vi "Initialize.vi"(8 "error in (no error)":errorcluster, 11 "UDPlog Thread User Interface in":refnum<class "UDPlog Thread User Interface.lvclass">) -> (0 "error out":errorcluster, 3 "UDPlog Thread User Interface out":refnum<class "UDPlog Thread User Interface.lvclass">)   [LabVIEW 2023, in "UDPlog.lvlib" / "UDPlog Thread User Interface.lvclass"]
uses:
  UDPlog Thread User Interface.lvclass
  C:/Users/Public/Documents/National Instruments/NI VeriStand 2023/Custom Devices/Data Sharing Framework/Linux_x64/DSF Core.lvlibp/Classes/User Interface/User Interface.lvclass
  Configurations/Thread/UDPlog Thread Configuration.lvclass
  C:/Users/Public/Documents/National Instruments/NI VeriStand 2023/Custom Devices/Data Sharing Framework/Linux_x64/DSF Core.lvlibp/Classes/Configuration/Configuration.lvclass
  Users/Public/Documents/National Instruments/NI VeriStand 2023/Custom Devices/Data Sharing Framework/Linux_x64/DSF Core.lvlibp/Classes/User Interface/User Interface.lvclass
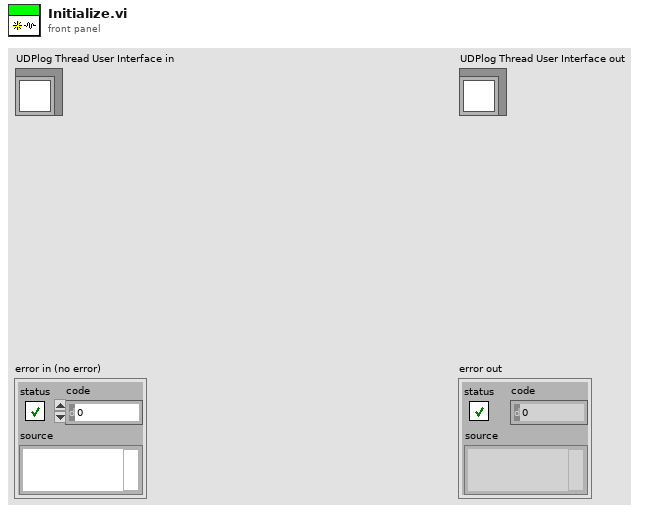
[diagram p1: front panel]
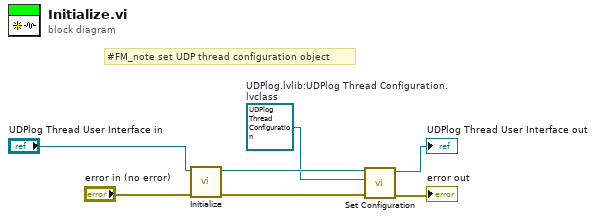
[diagram p0: block diagram]
diagram:
  w1 = refnum<class "UDPlog Thread Configuration.lvclass"> refnum  # UDPlog.lvlib:UDPlog Thread Configuration.lvclass
  # "#FM_note set UDP thread configuration object"
  n1 = call-parent "Initialize.vi"("error in (no error)"="error in (no error)", "User Interface in"="UDPlog Thread User Interface in") -> ("error out"=w5:errorcluster, "User Interface out"=w2:refnum<class "UDPlog Thread User Interface.lvclass">)  [unwired: 8 in]
  n2 = call "Set Configuration.vi"("error in (no error)"=w5, "configuration"=w1, "User Interface in"=w2) -> ("error out"=→"error out":errorcluster, "User Interface out"=→"UDPlog Thread User Interface out":refnum<class "UDPlog Thread User Interface.lvclass">)  [unwired: 7 in]
